vi "Write Library Name.vi"(8 "error in (no error)":errorcluster, 10 "Library Name":string, 11 "Library in":refnum<class "Library.lvclass">) -> (0 "error out":errorcluster, 3 "Library out":refnum<class "Library.lvclass">)   [LabVIEW 2019, in "Library.lvclass"]
uses:
  Library.lvclass
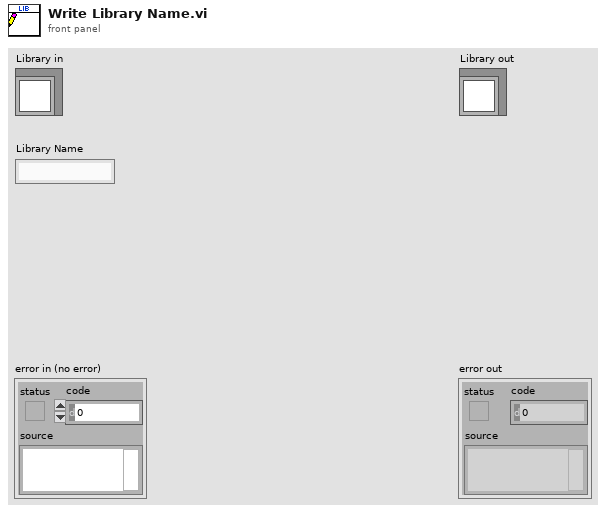
[diagram p1: front panel]
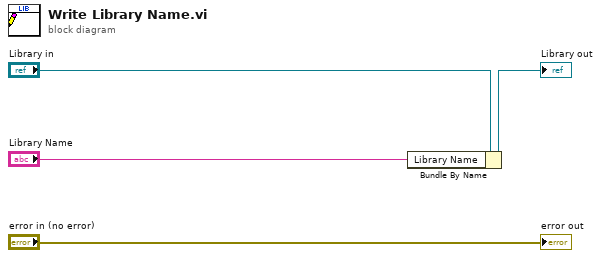
[diagram p0: block diagram]
diagram:
  n1 = Bundle By Name(cluster="Library in", "Library Name"="Library Name") -> (→"Library out":refnum<class "Library.lvclass">)
  "error out" <- "error in (no error)"
